vi "3-6.vi"() -> ()   [LabVIEW 2017]
panel:
  out "x*y":i8
  in  "Numeric":i8
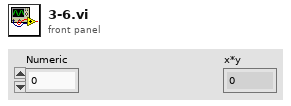
[diagram p1: front panel]
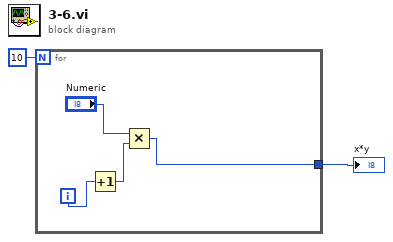
[diagram p0: block diagram]
diagram:
  n1 = for {
    N: 10 -> [_]
    tunnel: [w3] -> w1
    i -> [w5]
    n2 = Increment(x=w5) -> (x+1=w4:i32)
    n3 = Multiply(x="Numeric", y=w4) -> (x*y=w3:i32)
  }
  "x*y" <- w1
